vi "Initiate Powerup.vi"(0 "Instrument handles in":refnum<k15>[](array[refnum]), 5 "Channel Name":string[](array[string]), 11 "error in (no error)":errorcluster) -> (4 "Initiated?":bool[](array[boolean]), 15 "error out":errorcluster)   [LabVIEW 2024, in "devicePowerSequencerCoreLogic.lvlib"]
uses:
  devicePowerSequencerCoreLogic.lvlib
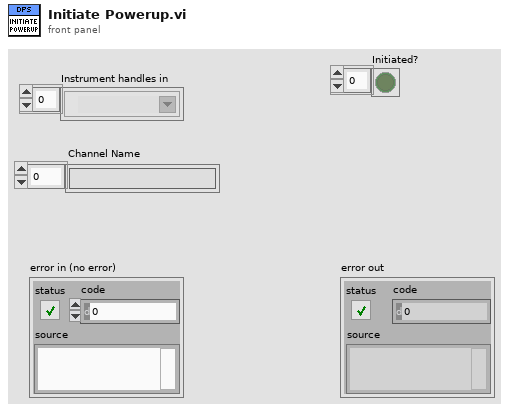
[diagram p1: front panel]
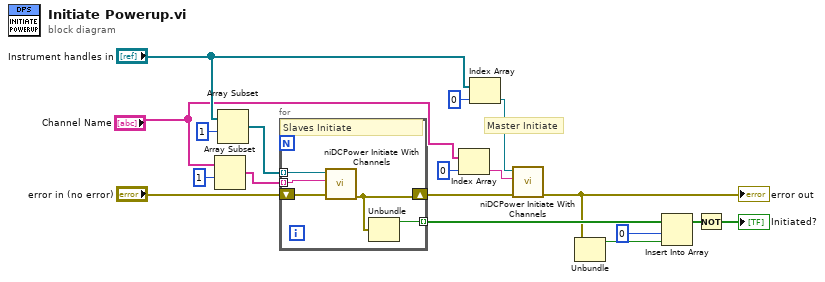
[diagram p0: block diagram]
diagram:
  # "Master Initiate"
  n1 = Array Subset(array="Channel Name", index=1) -> (w4:string[])  [unwired: 1 in]
  n2 = Array Subset(array="Instrument handles in", index=1) -> (w15:refnum<k15>[])  [unwired: 1 in]
  n3 = for {
    tunnel: w15 -> [w22] mode=indexing
    shift-right: [w21] -> w16
    shift-left: "error in (no error)" -> [w23]
    tunnel: [w20] -> w11 mode=indexing
    tunnel: w4 -> [w19] mode=indexing
    # "Slaves Initiate"
    n4 = call <instrlib>:"niDCPower Initiate With Channels.vi"("error in (no error)"=w23, "channel name"=w19, "instrument handle"=w22) -> ("error out"=w21:errorcluster)  [unwired: 7 in, 1 out]
    n5 = Unbundle(w21) -> ("status"=w20:bool)  [unwired: 2 out]
  }
  n6 = Index Array(array="Channel Name", index=0) -> (element=w1:string)
  n7 = Index Array(array="Instrument handles in", index=0) -> (element=w18:refnum<k15>)
  n8 = call <instrlib>:"niDCPower Initiate With Channels.vi"("error in (no error)"=w16, "channel name"=w1, "instrument handle"=w18) -> ("error out"=w9:errorcluster)  [unwired: 7 in, 1 out]
  "error out" <- w9
  n9 = Unbundle(w9) -> ("status"=w8:bool)  [unwired: 2 out]
  n10 = Insert Into Array(array=w11, index=0, new element=w8) -> (w7:bool[])
  n11 = Not(x=w7) -> (.not. x?=→"Initiated?":bool[])
